vi "timeInSeconds.vi"() -> (0 "Numeric":dbl, 1 "current time":timestamp)   [LabVIEW 2017]
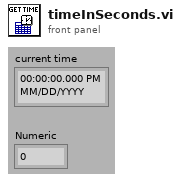
[diagram p1: front panel]
types:
  T1 = typedef "LVDateTimeRec.ctl" = cluster{"fractional second":dbl, "second":i32, "minute":i32, "hour":i32, "day of month":i32, "month":i32, "year":i32, "day of week":i32, "day of year":i32, "DST":i32}
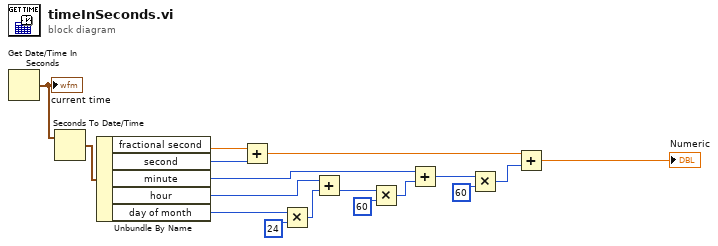
[diagram p0: block diagram]
diagram:
  n1 = Get Date/Time In Seconds() -> (seconds since 1Jan1904=w5:timestamp)
  "current time" <- w5
  n2 = Seconds To Date/Time(time stamp (now)=w5) -> (date time rec=w6:T1)  [unwired: 1 in]
  n3 = Unbundle By Name(w6) -> ("fractional second"=w8:dbl, "second"=w7:i32, "minute"=w9:i32, "hour"=w12:i32, "day of month"=w3:i32)
  n4 = Add(x=w8, y=w7) -> (x+y=w16:dbl)
  n5 = Multiply(x=w3, y=24) -> (x*y=w1:i32)
  n6 = Add(x=w12, y=w1) -> (x+y=w2:i32)
  n7 = Multiply(x=w2, y=60) -> (x*y=w14:i32)
  n8 = Add(x=w9, y=w14) -> (x+y=w13:i32)
  n9 = Multiply(x=w13, y=60) -> (x*y=w15:i32)
  n10 = Add(x=w16, y=w15) -> (x+y=→"Numeric":dbl)
